vi "Get Entity Paths.vi"(11 "Entity Path":path) -> (0 "error out":errorcluster, 3 "Entity Paths":T1)   [LabVIEW 2020, in "Conditum-Tools.lvlib" / "Entity Editor.lvclass"]
uses:
  Entity Editor.lvclass
  Entity Paths.ctl
  52e54c91-2e5b-4483-81c3-43126bd01008.vi
  41a8542e-d162-4a69-9911-75fba1b13349.vi
  Get Entity Paths OoC.vi
  Editor Context.vi
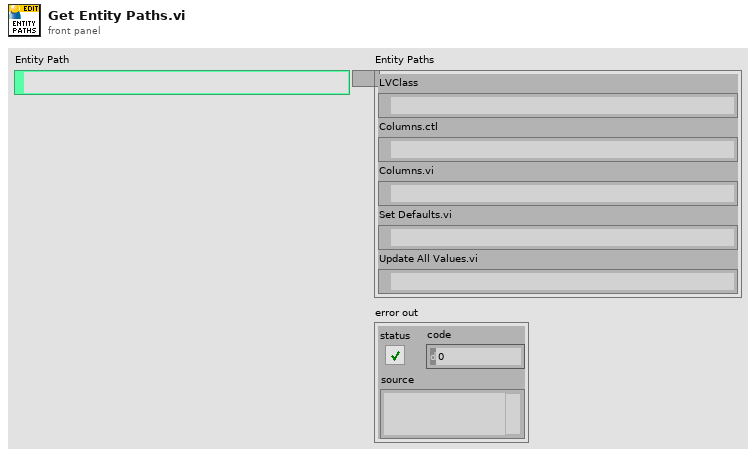
[diagram p1: front panel]
types:
  T1 = typedef "Conditum-Tools.lvlib/Entity Editor.lvclass/Entity Paths.ctl" = cluster{"LVClass":path, "Columns.ctl":path, "Columns.vi":path, "Set Defaults.vi":path, "Update All Values.vi":path}
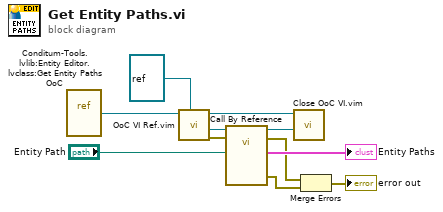
[diagram p0: block diagram]
diagram:
  n1 = vi-ref "Conditum-Tools.lvlib:Entity Editor.lvclass:Get Entity Paths OoC.vi"() -> (w7:refnum<vi>)
  n2 = call "OoC VI Ref.vim"("VI Type"=refnum<vi> refnum, "OoC SVR"=w7) -> ("error out"=w10:errorcluster, "vi reference"=w11:refnum<vi>, "context"=w9:refnum<vi>)  [unwired: 7 in]
  n3 = call-by-ref "?"(reference=w11, error in=w10, "Entity Path"="Entity Path") -> (reference out=w8:refnum<vi>, error out=w4:errorcluster, 0:"error out"=w3:errorcluster, "Entity Paths"=→"Entity Paths":T1)  [unwired: 9 in]
  n4 = call "Close OoC VI.vim"("vi reference"=w8, "context"=w9) -> ()  [unwired: 9 in, 1 out]
  n5 = Merge Errors(w4, w3) -> (→"error out":errorcluster)
